vi "Avg ILC Data.vi"(8 "error in (no error)":errorcluster, 9 "Before This Time":dbl, 10 "After This Time":dbl, 11 "Model in":refnum<class "Model.lvclass">) -> (0 "error out":errorcluster, 1 "Fy":dbl, 2 "Fz":dbl, 3 "Model out":refnum<class "Model.lvclass">)   [LabVIEW 2016, in "Model.lvclass"]
uses:
  Model.lvclass
  Model.lvclass/Model.ctl
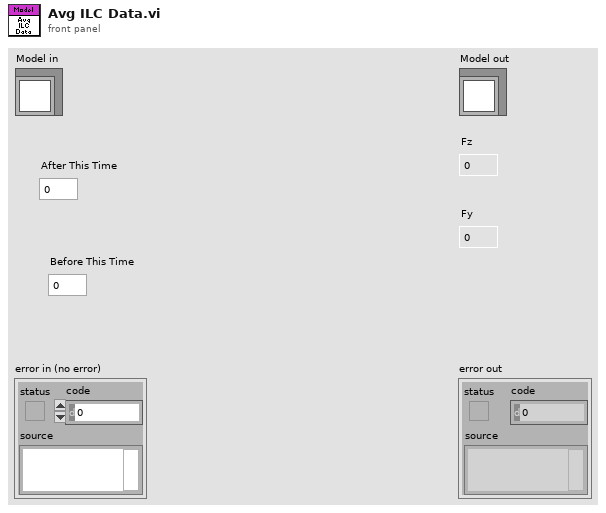
[diagram p1: front panel]
types:
  T1 = typedef "FAMT Typedefs.lvlib/ActuatorData.ctl" = cluster{"Timestamp":dbl, "Axial Force":dbl, "Lateral Force":dbl, "FC1 Force":dbl, "FC2 Force":dbl, "Lateral Push Pressure":dbl, "Lateral Pull Pressure":dbl, "Axial Push Pressure":dbl, "Axial Pull Pressure":dbl}
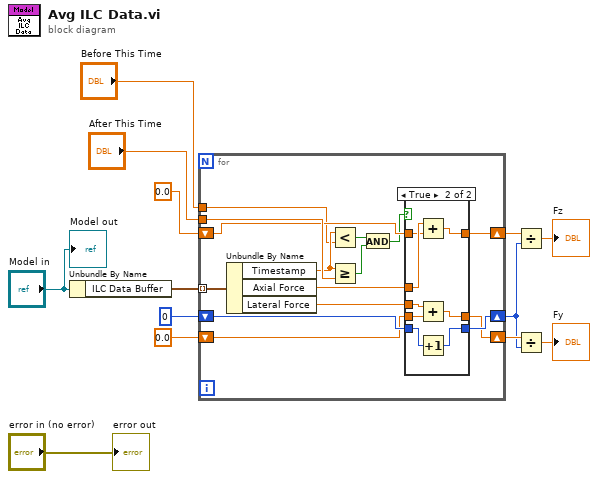
[diagram p0: block diagram]
diagram:
  n1 = Unbundle By Name("Model in") -> ("ILC Data Buffer"=w13:T1[])
  n2 = for {
    tunnel: w13 -> [w28] mode=indexing
    tunnel: "After This Time" -> [w27]
    shift-right: [w25] -> w8
    shift-left: 0.0 -> [w24]
    shift-right: [w22] -> w6
    shift-left: 0 -> [w23]
    shift-right: [w20] -> w7
    shift-left: 0.0 -> [w19]
    tunnel: "Before This Time" -> [w17]
    n3 = Unbundle By Name(w28) -> ("Timestamp"=w18:dbl, "Axial Force"=w26:dbl, "Lateral Force"=w21:dbl)
    n4 = Less?(x=w18, y=w17) -> (x < y?=w16:bool)
    n5 = Greater Or Equal?(x=w18, y=w27) -> (x >= y?=w15:bool)
    n6 = And(x=w16, y=w15) -> (x .and. y?=w14:bool)
    n7 = case shown="True" w14 {
      tunnel: w26 -> [_ w39]
      tunnel: [w30 w38] -> w25
      tunnel: w24 -> [w30 w37]
      tunnel: w23 -> [w31 w36]
      tunnel: [w31 w35] -> w22
      tunnel: w21 -> [_ w34]
      tunnel: [w29 w33] -> w20
      tunnel: w19 -> [w29 w32]
      frame False {
      }
      frame True {
        n8 = Add(x=w39, y=w37) -> (x+y=w38:dbl)
        n9 = Add(x=w34, y=w32) -> (x+y=w33:dbl)
        n10 = Increment(x=w36) -> (x+1=w35:i32)
      }
    }
  }
  n11 = Divide(x=w8, y=w6) -> (x/y=→"Fz":dbl)
  n12 = Divide(x=w7, y=w6) -> (x/y=→"Fy":dbl)
  "error out" <- "error in (no error)"
  "Model out" <- "Model in"
